vi "post-reaction-test-simple.vi"() -> ()   [LabVIEW 2023]
uses:
  <vilib>/DAQmx/read.llb/DAQmx Read (Digital 1D Bool 1Chan 1Samp).vi
  <vilib>/DAQmx/create/channels.llb/DAQmx Create Channel (DI-Digital Input).vi
  <vilib>/DAQmx/miscellaneous.llb/DAQmx Fill In Error Info.vi
panel:
  in  "IS Volume (μL)":u16=20
  out "sensor":bool[](array[boolean])
  in  "stop":bool
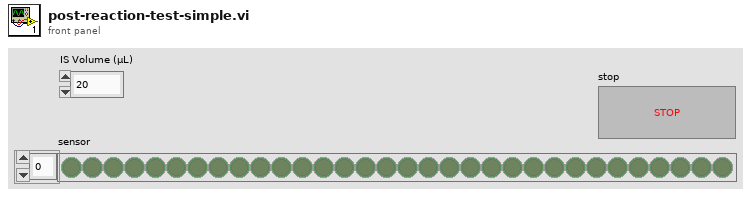
[diagram p1: front panel]
types:
  T1 = enum16{"Initialize", "Absolute Position", "Relative Pickup", "Relative Dispense", "Swich valve", "Bypass"}
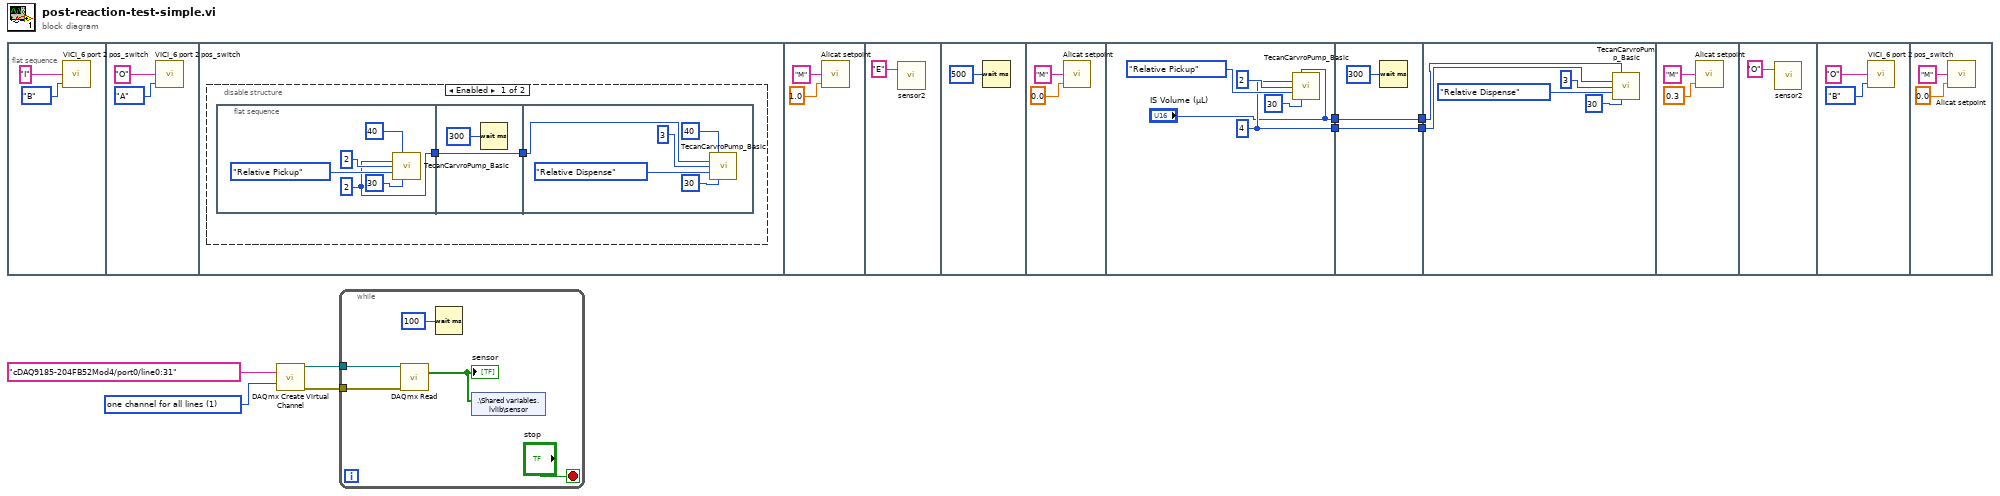
[diagram p0: block diagram]
diagram:
  w8 = 1 items=["one channel for each line", "one channel for all lines"] ("line grouping")
  n1 = flat-sequence {
    tunnel: [w34] -> w3
    tunnel: ["IS Volume (μL)"] -> w1
    tunnel: [w39] -> w4
    tunnel: w3 -> [w39]
    tunnel: [w38] -> w2
    tunnel: w1 -> [w38]
    tunnel: w4 -> [w42]
    tunnel: w2 -> [w41]
    frame #0 {
      n2 = call "VICI_6 port 2 pos_switch.vi"("Switch to position (A/B)"=enum16{"A", "B"}."B", "Valve ID"="I") -> ()  [unwired: 2 in, 1 out]
    }
    frame #1 {
      n3 = call "VICI_6 port 2 pos_switch.vi"("Switch to position (A/B)"=enum16{"A", "B"}."A", "Valve ID"="O") -> ()  [unwired: 2 in, 1 out]
    }
    frame #2 {
      n4 = disable-structure shown="Enabled" {
        frame Enabled {
          n5 = flat-sequence {
            tunnel: [w15] -> w14
            tunnel: w14 -> [w21]
            tunnel: [w21] -> w13
            tunnel: w13 -> [w22]
            frame #0 {
              w15 = u8 2 ("TecanPump address")
              n6 = call "TecanCarvroPump_Basic.vi"("Volume (μL)"=u16 40, "TecanPump address"=w15, "Valve"=u8 2, "Mode"=T1."Relative Pickup", "Speed (μL/s)"=u16 30) -> ()  [unwired: 10 in, 1 out]
            }
            frame #1 {
              n7 = Wait (ms)(milliseconds to wait=u32 300) -> ()  [unwired: 1 out]
            }
            frame #2 {
              n8 = call "TecanCarvroPump_Basic.vi"("Volume (μL)"=u16 40, "TecanPump address"=w22, "Valve"=u8 3, "Mode"=T1."Relative Dispense", "Speed (μL/s)"=u16 30) -> ()  [unwired: 10 in, 1 out]
            }
          }
        }
        frame Disabled {
        }
      }
    }
    frame #3 {
      n9 = call "Alicat setpoint.vi"("Setpoint"=1.0, "Unit ID"="M") -> ()  [unwired: 3 in]
    }
    frame #4 {
      n10 = call "sensor2.vi"("Sensor"="E") -> ()  [unwired: 1 in, 2 out]
    }
    frame #5 {
      n11 = Wait (ms)(milliseconds to wait=u32 500) -> ()  [unwired: 1 out]
    }
    frame #6 {
      n12 = call "Alicat setpoint.vi"("Setpoint"=0.0, "Unit ID"="M") -> ()  [unwired: 3 in]
    }
    frame #7 {
      w34 = u8 4 ("TecanPump address")
      n13 = call "TecanCarvroPump_Basic.vi"("Volume (μL)"="IS Volume (μL)", "TecanPump address"=w34, "Valve"=u8 2, "Mode"=T1."Relative Pickup", "Speed (μL/s)"=u16 30) -> ()  [unwired: 10 in, 1 out]
    }
    frame #8 {
      n14 = Wait (ms)(milliseconds to wait=u32 300) -> ()  [unwired: 1 out]
    }
    frame #9 {
      n15 = call "TecanCarvroPump_Basic.vi"("Volume (μL)"=w41, "TecanPump address"=w42, "Valve"=u8 3, "Mode"=T1."Relative Dispense", "Speed (μL/s)"=u16 30) -> ()  [unwired: 10 in, 1 out]
    }
    frame #10 {
      n16 = call "Alicat setpoint.vi"("Setpoint"=0.3, "Unit ID"="M") -> ()  [unwired: 3 in]
    }
    frame #11 {
      n17 = call "sensor2.vi"("Sensor"="O") -> ()  [unwired: 1 in, 2 out]
    }
    frame #12 {
      n18 = call "VICI_6 port 2 pos_switch.vi"("Switch to position (A/B)"=enum16{"A", "B"}."B", "Valve ID"="O") -> ()  [unwired: 2 in, 1 out]
    }
    frame #13 {
      n19 = call "Alicat setpoint.vi"("Setpoint"=0.0, "Unit ID"="M") -> ()  [unwired: 3 in]
    }
  }
  n20 = call-poly <vilib>:"DAQmx Create Virtual Channel.vi"("lines"=tag "cDAQ9185-204FB52Mod4/port0/line0:31", "line grouping"=w8) -> ("task out"=w7:refnum<k21>, "error out"=w6:errorcluster)  [unwired: 12 in]
  n21 = while {
    tunnel: w7 -> [w57]
    tunnel: w6 -> [w56]
    stop <- "stop" stop-if-true
    n22 = call-poly <vilib>:"DAQmx Read.vi"("task/channels in"=w57, "error in"=w56) -> ("data"=w55:bool[])  [unwired: 11 in, 2 out]
    "sensor" <- w55
    n23 = Wait (ms)(milliseconds to wait=u32 100) -> ()  [unwired: 1 out]
    n24 = shared-variable ".\\Shared variables.lvlib\\sensor"(w55) -> ()  [unwired: 1 in, 1 out]
  }
